vi "New.vi"(11 "BlueJSONTextSerializer":refnum<class "BlueJSONTextSerializer.lvclass">) -> (3 "BlueJSONtext LVClass Serializer out":refnum<class "BlueJSONtext LVClass Serializer.lvclass">)   [LabVIEW 2019, in "BlueJSONTextSerializer.lvlib" / "BlueJSONtext LVClass Serializer.lvclass"]
uses:
  BlueJSONtext LVClass Serializer.lvclass
  BlueJSONTextSerializer/BlueJSONTextSerializer.lvclass
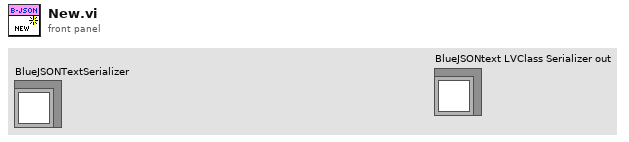
[diagram p1: front panel]
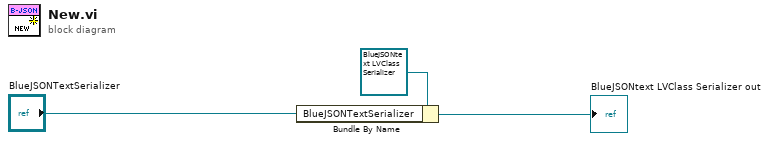
[diagram p0: block diagram]
diagram:
  n1 = Bundle By Name(cluster=refnum<class "BlueJSONtext LVClass Serializer.lvclass"> refnum ("BlueJSONtext LVClass Serializer in"), "BlueJSONTextSerializer"="BlueJSONTextSerializer") -> (→"BlueJSONtext LVClass Serializer out":refnum<class "BlueJSONtext LVClass Serializer.lvclass">)
